vi "Calculate.vi"(8 "error in (no error)":errorcluster, 10 "X":i64, 11 "Trace in":refnum<class "Trace.lvclass">) -> (0 "error out":errorcluster, 2 "Y":refnum<class "High Res Arithmetic.lvclass">, 3 "Trace out":refnum<class "Trace.lvclass">)   [LabVIEW 2021, in "Trace.lvclass"]
uses:
  Trace.lvclass
  High Res Arithmetic/High Res Arithmetic.lvclass
  Trace.lvclass/Trace.ctl
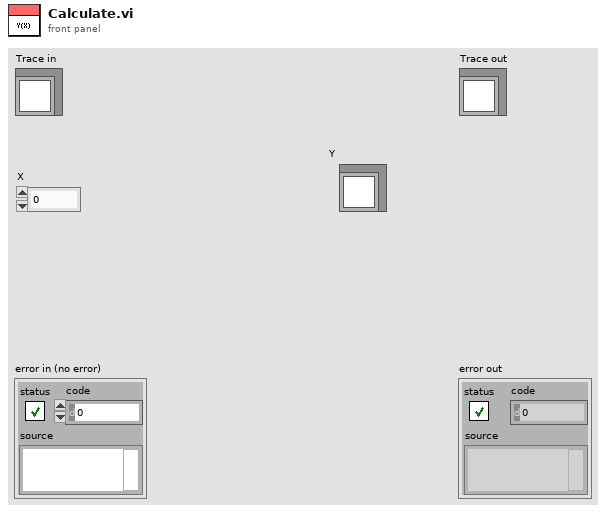
[diagram p1: front panel]
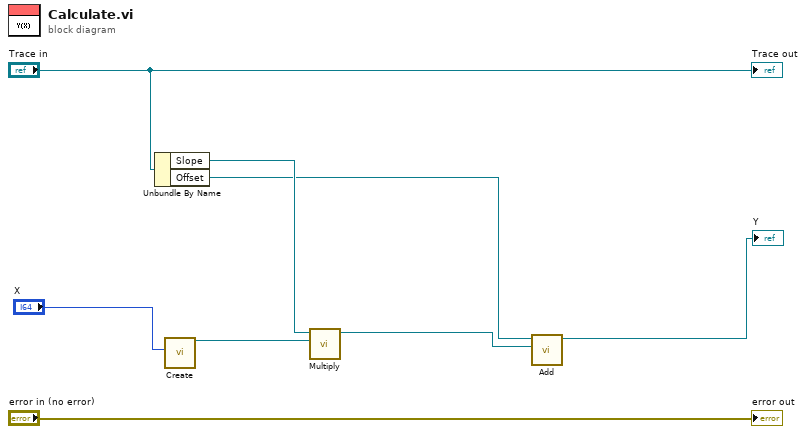
[diagram p0: block diagram]
diagram:
  n1 = Unbundle By Name("Trace in") -> ("Slope"=w4:refnum<class "High Res Arithmetic.lvclass">, "Offset"=w2:refnum<class "High Res Arithmetic.lvclass">)
  n2 = call "Create.vi"("Numerator"="X") -> ("Hi Res Arithm Test"=w5:refnum<class "High Res Arithmetic.lvclass">)  [unwired: 9 in, 1 out]
  n3 = call "Multiply.vi"("High Res Arithmetic 2"=w5, "High Res Arithmetic 1"=w4) -> ("High Res Arithmetic sum"=w3:refnum<class "High Res Arithmetic.lvclass">)  [unwired: 8 in, 1 out]
  n4 = call "Add.vi"("High Res Arithmetic 2"=w3, "High Res Arithmetic 1"=w2) -> ("High Res Arithmetic sum"=→"Y":refnum<class "High Res Arithmetic.lvclass">)  [unwired: 8 in, 1 out]
  "error out" <- "error in (no error)"
  "Trace out" <- "Trace in"
